vi "Configure Setpoint (Direct).vi"(8 "error in (no error)":errorcluster, 9 "Setpoint Direct (0)":sgl min=0 step=1 format="%#_5g", 10 "Node (3)":u8=3 caption="Node" min=3 max=128 step=1, 11 "VISA resource name":refnum<visa-resource-name>) -> (0 "error out":errorcluster, 3 "VISA resource name out":refnum<visa-resource-name>)   [LabVIEW 2024, in "Bronkhorst FLOW-BUS.lvlib"]
doc: "Configures the setpoint value in the instrument. The setpoint is used to tell the PID controller in the instrument what the wanted amount of mass flow or pressure is."
uses:
  Bronkhorst FLOW-BUS.lvlib
  Private/FLOW-BUS RW.ctl
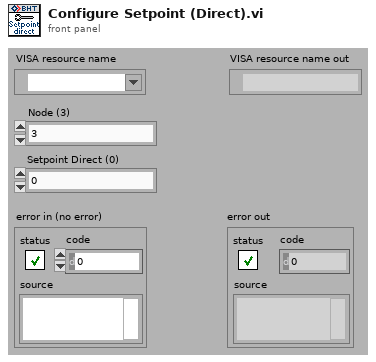
[diagram p1: front panel]
types:
  T1 = typedef "Bronkhorst FLOW-BUS.lvlib/FLOW-BUS RW.ctl" = cluster{"Node Address (3)":u8, "Communication Command":enum16{"Status message", "Send parameter with destination address and 00 response", "Send parameter with destination address", "Request parameter"}, "Process (0)":u16, "Parameter (0)":u16, "Data Type (0: Character)":enum16{"Character", "Integer", "Float or Long", "String"}, "Data for Char, Int, or Long (0)":u32, "Data for Float (0)":sgl, "Data for String":string, "Length of Requested String (0)":u8}
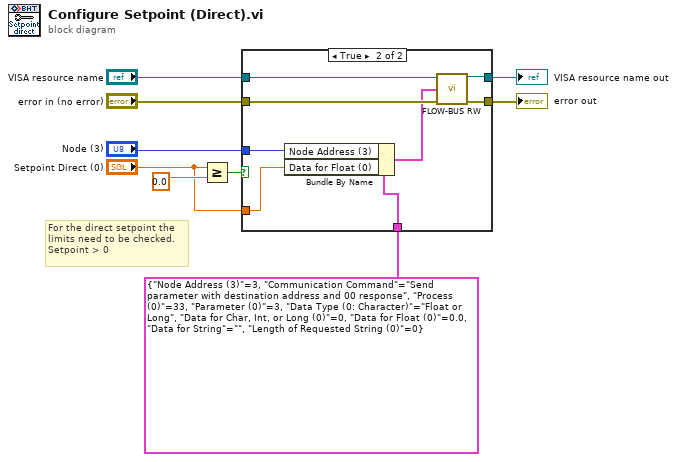
[diagram p0: block diagram]
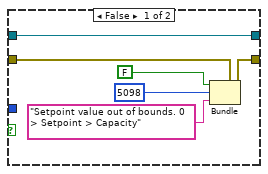
[diagram p2: hidden frame]
diagram:
  # "For the direct setpoint the \nlimits need to be checked.\nSetpoint > 0"
  n1 = Greater Or Equal?(x="Setpoint Direct (0)", y=sgl 0.0) -> (x >= y?=w4:bool)
  n2 = case shown="True" w4 {
    tunnel: [w15 w18] -> w7
    tunnel: "VISA resource name" -> [w15 w20]
    tunnel: "error in (no error)" -> [w12 w19]
    tunnel: "Setpoint Direct (0)" -> [_ w22]
    tunnel: "Node (3)" -> [_ w21]
    tunnel: [w11 w17] -> w6
    tunnel: T1 {"Node Address (3)"=3, "Communication Command"=enum."Send parameter with destination address and 00 response", "Process (0)"=33, "Parameter (0)"=3, "Data Type (0: Character)"=enum."Float or Long", "Data for Char, Int, or Long (0)"=0, "Data for Float (0)"=0.0, "Data for String"="", "Length of Requested String (0)"=0} ("FLOW-BUS Command Settings") -> [_ w23]
    frame False {
      n3 = Bundle(cluster=w12, "status"=FALSE, "code"=5098, "source"="Setpoint value out of bounds. 0 > Setpoint > Capacity") -> (w11:errorcluster)
    }
    frame True {
      n4 = Bundle By Name(cluster=w23, "Node Address (3)"=w21, "Data for Float (0)"=w22) -> (w16:T1)
      n5 = call "FLOW-BUS RW.vi"("VISA resource name"=w20, "FLOW-BUS Command Settings"=w16, "error in (no error)"=w19) -> ("VISA resource name out"=w18:refnum<visa-resource-name>, "error out"=w17:errorcluster)  [unwired: 8 in, 3 out]
    }
  }
  "VISA resource name out" <- w7
  "error out" <- w6
